vi "Init.vi"(8 "error in (no error)":errorcluster, 11 "Initial String (Empty)":string) -> (0 "error out":errorcluster, 3 "StringStream out":refnum<class "StringStream.lvclass">)   [LabVIEW 2020, in "Stream.lvlib" / "StringStream.lvclass"]
uses:
  StringStream.lvclass
  C:/dev/illuminated-g/lv-stream/stream/Stream/Stream.lvclass
  Ref Data.ctl
  StringStream.lvclass/StringStream.ctl
  Stream/Stream.lvclass
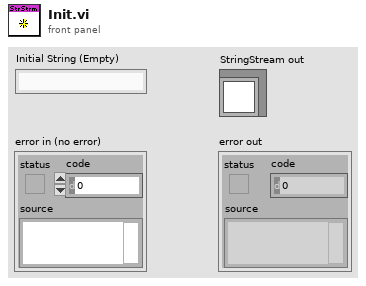
[diagram p1: front panel]
types:
  T1 = typedef "Stream.lvlib/StringStream.lvclass/Ref Data.ctl" = cluster{"Position":i64, "String":string}
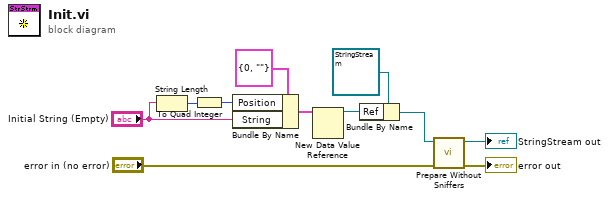
[diagram p0: block diagram]
diagram:
  n1 = String Length(string="Initial String (Empty)") -> (length=w9:i32)
  n2 = To Quad Integer(1:w9) -> (0:w7:i64)
  n3 = Bundle By Name(cluster=T1 {"Position"=0, "String"=""} ("Ref Data"), "Position"=w7, "String"="Initial String (Empty)") -> (w6:T1)
  n4 = New Data Value Reference(data value=w6) -> (data value reference=w5:refnum<data-value>)  [unwired: 1 in, 1 out]
  n5 = Bundle By Name(cluster=refnum<class "StringStream.lvclass"> refnum ("StringStream in"), "Ref"=w5) -> (w3:refnum<class "StringStream.lvclass">)
  n6 = call "Prepare Without Sniffers.vi"("error in (no error)"="error in (no error)", "Stream in"=w3) -> ("error out"=→"error out":errorcluster, "Stream out"=→"StringStream out":refnum<class "StringStream.lvclass">)  [unwired: 8 in]
